vi "CRYAPI Model Open GraphWindow.vi"(9 "sOption":string, 10 "sData":string) -> (0 "nID":i32, 3 "cView_Out":T1)   [LabVIEW 2013]
uses:
  CRYMain Sub Window Global.vi
  DataView/VIEW/CRYNew View Global.vi
  DataView/VIEW/CRYView Global.vi
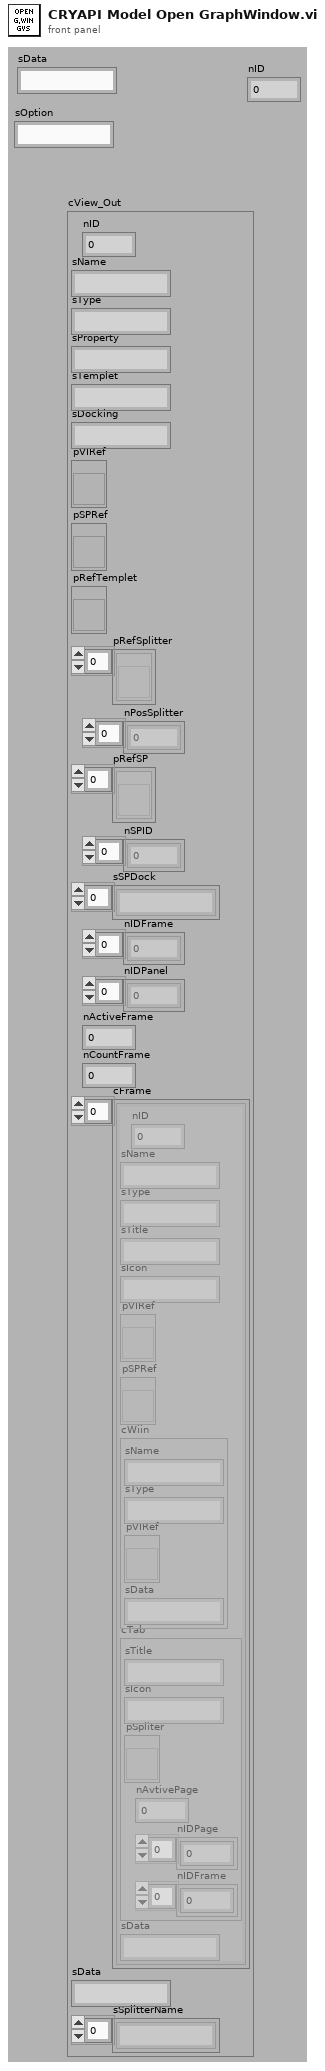
[diagram p1: front panel]
types:
  T1 = cluster{"nID":i32, "sName":string, "sType":string, "sProperty":string, "sTemplet":string, "sDocking":string, "pVIRef":refnum<vi>, "pSPRef":refnum<vi>, "pRefTemplet":refnum<vi>, "pRefSplitter":refnum<vi>[], "nPosSplitter":i32[], "pRefSP":refnum<vi>[], "nSPID":i32[], "sSPDock":string[], "nIDFrame":i32[], "nIDPanel":i32[], "nActiveFrame":i32, "nCountFrame":i32, "cFrame":cluster{"nID":i32, "sName":string, "sType":string, "sTitle":string, "sIcon":string, "pVIRef":refnum<vi>, "pSPRef":refnum<vi>, "cWiin":cluster{"sName":string, "sType":string, "pVIRef":refnum<vi>, "sData":string}, "cTab":cluster{"sTitle":string, "sIcon":string, "pSpliter":refnum<vi>, "nAvtivePage":i32, "nIDPage":i32[], "nIDFrame":i32[]}, "sData":string}[], "sData":string, "sSplitterName":string[]}
  T2 = typedef "Graph Main Info Cluster.ctl" = cluster{"Selected_BarIdx":i32, "Selected_PanelIdx":i32, "Graph Main VIRef":refnum<vi>, "ToolBarClick":bool, "Spliter Ref Array":refnum<vi>[], "Panel Ref Array":refnum<vi>[], "Spliter_matrix":i32[][], "Panel_matrix":i32[][], "child_spliterIdx_matrix":i32[][], "split_pos_matrix":i32[][], "Title State":bool, "sQueueName":string, "Frame nID":i32, "Graph VIRef Array":cluster{"Graph VIRef":refnum<vi>, "Panel Idx":i32, "Frame VIRef":refnum<vi>, "Icon Ring":i32, "Graph Type":string}[], "View Type":string}
  T3 = typedef "LVRectTypeDef.ctl" = cluster{"Left":i16, "Top":i16, "Right":i16, "Bottom":i16}
  T4 = cluster{"nType":i32, "nParent":i32, "pVIW":refnum<vi>, "pSPW":refnum<vi>, "nTypeF":i32, "pVIF":refnum<vi>, "pSPF":refnum<vi>, "nIDSpliter":i32, "nProperty":i32, "Bound":T3, "nID":i32, "nData":i32, "sData":string, "pWVI":refnum<vi>, "sTitle":string, "cPages":cluster{"nPage":i32, "sTitle":string, "sIcon":string, "pVI":refnum<vi>, "nID":i32}[], "pTab":refnum<vi>, "nIDPages":i32[], "pSPT":refnum<vi>, "sTemp":string, "nDockID":i32, "nDockLR":i32, "sIcon":string}
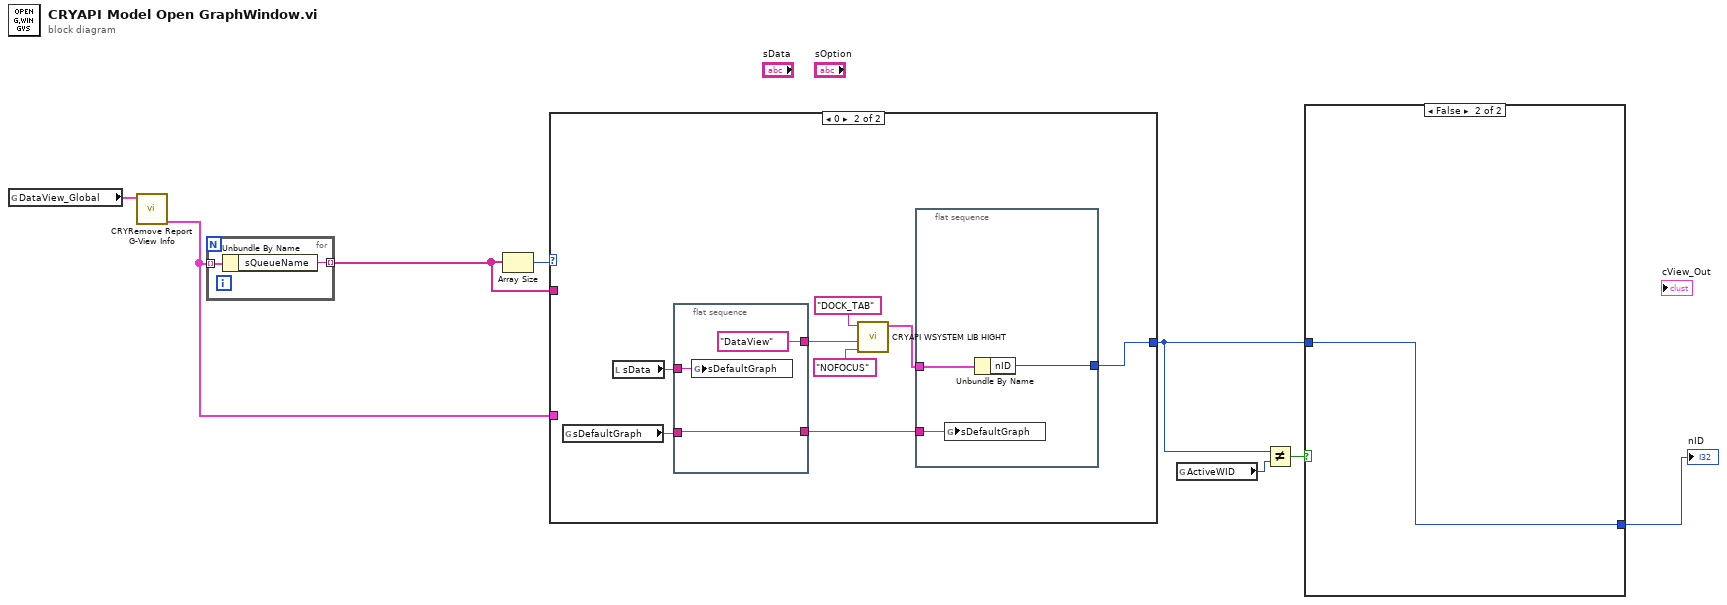
[diagram p0: block diagram]
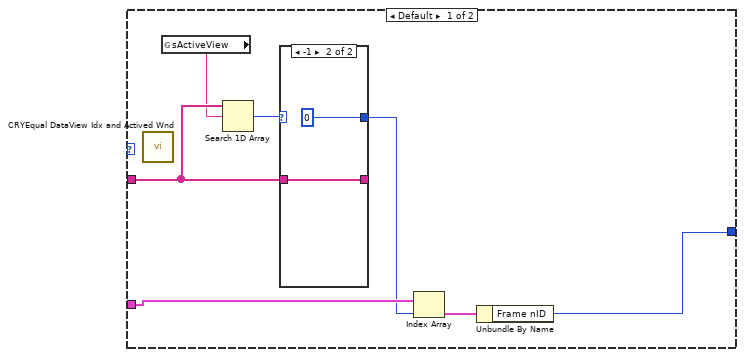
[diagram p2: hidden frame]
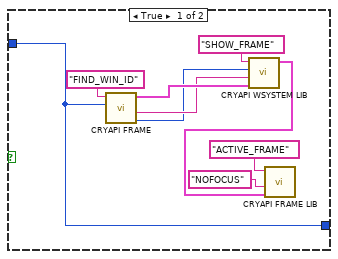
[diagram p4: hidden frame]
diagram:
  n1 = global read "CRYNew View Global.vi" "DataView_Global"() -> (w2:T2[])
  n2 = call "CRYRemove Report G-View Info.vi"("DataView_Info Array"=w2) -> ("DataView_Info Array Except Report out"=w1:T2[])  [unwired: 9 in, 1 out]
  n3 = for {
    tunnel: w1 -> [w10] mode=indexing
    tunnel: [w9] -> w4 mode=indexing
    n4 = Unbundle By Name(w10) -> ("sQueueName"=w9:string)
  }
  n5 = Array Size(array=w4) -> (size(s)=w6:i32)
  n6 = case shown="0" w6 {
    tunnel: w4 -> [w17 _]
    tunnel: [w12 w22] -> w5
    tunnel: w1 -> [w15 _]
    frame Default {
      n7 = call "CRYEqual DataView Idx and Actived Wnd.vi"() -> ()  [unwired: 9 in, 3 out]
      n8 = global read "CRYView Global.vi" "sActiveView"() -> (w11:string)
      n9 = Search 1D Array(1D array=w17, element=w11) -> (index of element=w16:i32)  [unwired: 1 in]
      n10 = case shown="-1" w16 {
        selector: w16 -> [w19 _]
        tunnel: w17 -> [w18 w20]
        tunnel: [w19 0] -> w14
        tunnel: [w18 w20] -> _
        frame Default {
        }
        frame -1 {
        }
      }
      n11 = Index Array(array=w15, index=w14) -> (element=w13:T2)
      n12 = Unbundle By Name(w13) -> ("Frame nID"=w12:i32)
    }
    frame 0 {
      n13 = global read "CRYView Global.vi" "sDefaultGraph"() -> (w24:string)
      n14 = local read "sData"() -> (w25:string)
      n15 = flat-sequence {
        tunnel: ["DataView" ("Window Type")] -> w28
        tunnel: [w34] -> w29
        tunnel: w25 -> [w33]
        tunnel: w24 -> [w34]
        frame #0 {
          n16 = global write "CRYView Global.vi" "sDefaultGraph"(w33) -> ()
        }
      }
      n17 = call "CRYAPI WSYSTEM LIB HIGHT.vi"("sOption"="NOFOCUS", "sData"=w28, "sAction"="DOCK_TAB") -> ("tFrame_Out"=w23:T4)  [unwired: 1 in, 7 out]
      n18 = flat-sequence {
        tunnel: w29 -> [w32]
        tunnel: w23 -> [w31]
        tunnel: [w30] -> w22
        frame #0 {
          n19 = global write "CRYView Global.vi" "sDefaultGraph"(w32) -> ()
          n20 = Unbundle By Name(w31) -> ("nID"=w30:i32)
        }
      }
    }
  }
  n21 = global read "CRYMain Sub Window Global.vi" "ActiveWID"() -> (w8:i32)
  n22 = Not Equal?(x=w5, y=w8) -> (x != y?=w7:bool)
  n23 = case shown="False" w7 {
    tunnel: w5 -> [w36 w45]
    tunnel: [w36 w45] -> w3
    frame True {
      n24 = call "CRYAPI FRAME.vi"("nData"=w36, "sAction"="FIND_WIN_ID") -> ("nData_Out"=w40:i32, "sData_Out"=w41:string, "tFrame_Out"=w42:T4)  [unwired: 4 in, 3 out]
      n25 = call "CRYAPI WSYSTEM LIB.vi"("tFrame"=w42, "sData"=w41, "nData"=w40, "sAction"="SHOW_FRAME") -> ("tFrame_Out"=w44:T4)  [unwired: 7 out]
      n26 = call "CRYAPI FRAME LIB.vi"("tFrame"=w44, "sData"="NOFOCUS", "sAction"="ACTIVE_FRAME") -> ()  [unwired: 3 in, 6 out]
    }
    frame False {
    }
  }
  "nID" <- w3
